vi "Vertex.vi"(4 "Radius":sgl=0.01, 5 "Font Size":sgl, 6 "Vertex label?":bool, 7 "Color":T1={"Red"=1.0, "Green"=0.0, "Blue"=0.0, "Alpha"=1.0}, 8 "error in (no error)":errorcluster, 9 "Length":sgl=2.0 step=0.01, 10 "Enum":enum16{"X Axis", "Y Axis", "Z Axis"}(ring), 11 "Name":string="XYZ axis") -> (0 "error out":errorcluster, 3 "New Object Refnum":refnum<vi>)   [LabVIEW 2021]
uses:
  <vilib>/Utility/miscctls.llb/LVSceneTextAlignment.ctl
  <vilib>/picture/3D Picture Control/Object/Create Object (name).vi
  <vilib>/picture/3D Picture Control/Object/Create Object (drawable).vi
  <vilib>/picture/3D Picture Control/Object/Add Object (no reference).vi
  <vilib>/picture/3D Picture Control/NI_3D Picture Control.lvlib
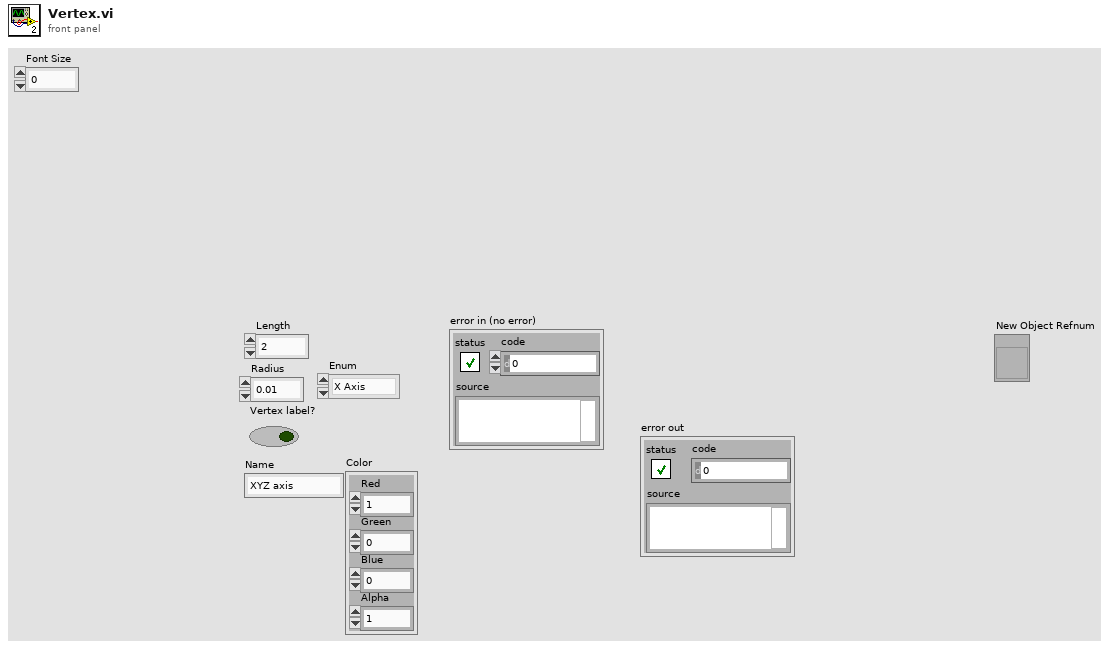
[diagram p1: front panel]
types:
  T1 = cluster{"Red":sgl, "Green":sgl, "Blue":sgl, "Alpha":sgl}
  T2 = typedef "LVSceneTextAlignment.ctl" = cluster{"Horizontal Alignment":enum8{"Left", "Right", "Center"}, "Vertical Alignment":enum8{"Top", "Bottom", "Center", "Base Line", "Bottom Base Line"}}
  T3 = cluster{"Alignment":T2, "Axis Alignment":enum8{"X-Y", "Y-Z", "X-Z", "Reversed X-Y", "Reversed Y-Z", "Reversed X-Z", "Screen"}, "Vertical?":bool, "Wrap Distance":sgl}
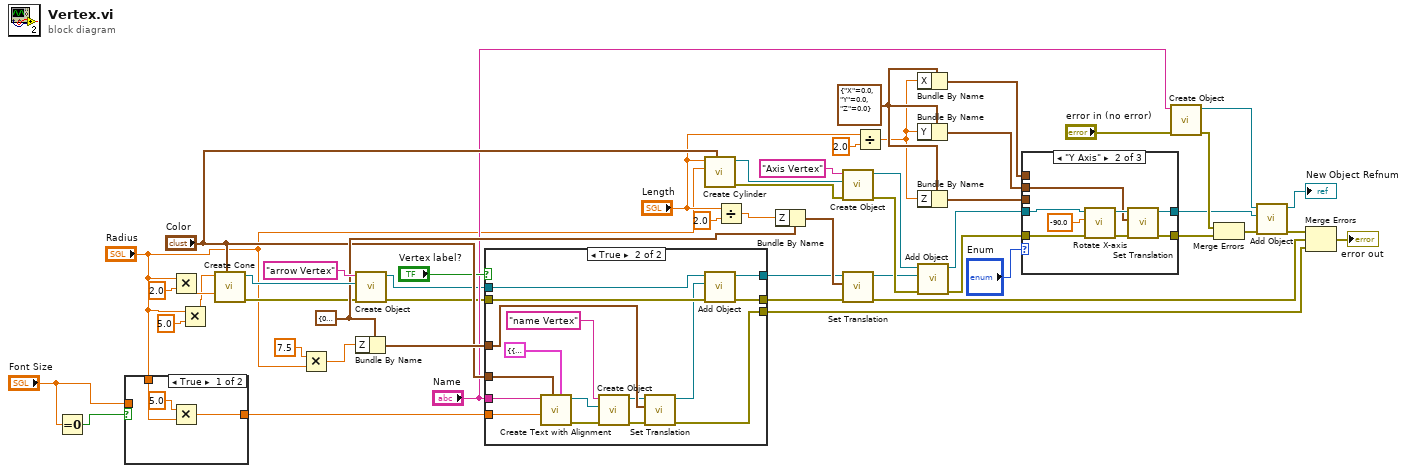
[diagram p0: block diagram]
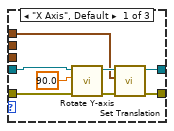
[diagram p3: hidden frame]
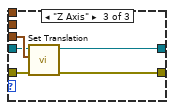
[diagram p4: hidden frame]
diagram:
  w40 = cluster{"X":sgl, "Y":sgl, "Z":sgl} {"X"=0.0, "Y"=0.0, "Z"=0.0} ("Translation")
  w38 = cluster{"X":sgl, "Y":sgl, "Z":sgl} {"X"=0.0, "Y"=0.0, "Z"=0.0} ("Translation")
  n1 = Equal To 0?(x="Font Size") -> (x = 0?=w5:bool)
  n2 = case shown="True" w5 {
    tunnel: "Radius" -> [w54 _]
    tunnel: [w53 w56] -> w7
    tunnel: "Font Size" -> [_ w56]
    frame True {
      n3 = Multiply(x=sgl 5.0 ("y"), y=w54) -> (x*y=w53:sgl)
    }
    frame False {
    }
  }
  n4 = Multiply(x="Radius", y=sgl 2.0) -> (x*y=w4:sgl)
  n5 = Multiply(x="Radius", y=sgl 5.0) -> (x*y=w1:sgl)
  n6 = call <vilib>:"Create Cone.vi"("Color"="Color", "Radius"=w4, "Height"=w1) -> ("error out"=w36:errorcluster, "New Cone Refnum"=w41:refnum<vi>)  [unwired: 7 in]
  n7 = Multiply(x=sgl 7.5 ("y"), y="Radius") -> (x*y=w8:sgl)
  n8 = call-poly <vilib>:"Create Object.vi"("error in (no error)"=w36, "Geometry"=w41, "Name"="arrow Vertex") -> ("error out"=w11:errorcluster, "Scene:New Object"=w10:refnum<vi>)  [unwired: 7 in]
  n9 = Bundle By Name(cluster=w38, "Z"=w8) -> (w37:cluster{"X":sgl, "Y":sgl, "Z":sgl})
  n10 = case shown="True" "Vertex label?" {
    tunnel: [w58 w74] -> w14
    tunnel: w37 -> [_ w73]
    tunnel: [w57 w72] -> w13
    tunnel: [_ w65] -> w28
    tunnel: "Color" -> [_ w71]
    tunnel: w7 -> [_ w66]
    tunnel: "Name" -> [_ w64]
    tunnel: w11 -> [w57 w62]
    tunnel: w10 -> [w58 w61]
    frame False {
    }
    frame True {
      n11 = call <vilib>:"Create Text with Alignment.vi"("Font Options"=T3 {"Alignment"={"Horizontal Alignment"=enum."Center", "Vertical Alignment"=enum."Center"}, "Axis Alignment"=enum."Screen", "Vertical?"=FALSE, "Wrap Distance"=0.0} ("Font options"), "Color"=w71, "Character Size"=w66, "Text"=w64) -> ("error out"=w67:errorcluster, "New Text Refnum"=w70:refnum<vi>)  [unwired: 6 in]
      n12 = call-poly <vilib>:"Create Object.vi"("error in (no error)"=w67, "Geometry"=w70, "Name"="name Vertex") -> ("error out"=w68:errorcluster, "Scene:New Object"=w69:refnum<vi>)  [unwired: 7 in]
      n13 = call <vilib>:"Set Translation.vi"("error in (no error)"=w68, "Translation"=w73, "Scene Object"=w69) -> ("error out"=w65:errorcluster, "Translated Object"=w60:refnum<vi>)  [unwired: 7 in]
      n14 = call-poly <vilib>:"Add Object.vi"("error in (no error)"=w62, "New Object In"=w60, "Scene Object In"=w61) -> ("error out"=w72:errorcluster, "Scene Object Out"=w74:refnum<vi>)  [unwired: 7 in]
    }
  }
  n15 = call <vilib>:"Create Cylinder.vi"("Color"="Color", "Radius"="Radius", "Height"="Length") -> ("error out"=w48:errorcluster, "New Cylinder Refnum"=w51:refnum<vi>)  [unwired: 7 in]
  n16 = Divide(x="Length", y=sgl 2.0 ("x")) -> (x/y=w35:sgl)
  n17 = Bundle By Name(cluster=w38, "Z"=w35) -> (w16:cluster{"X":sgl, "Y":sgl, "Z":sgl})
  n18 = call-poly <vilib>:"Create Object.vi"("error in (no error)"=w48, "Geometry"=w51, "Name"="Axis Vertex") -> ("error out"=w22:errorcluster, "Scene:New Object"=w21:refnum<vi>)  [unwired: 7 in]
  n19 = call <vilib>:"Set Translation.vi"("error in (no error)"=w13, "Translation"=w16, "Scene Object"=w14) -> ("error out"=w12:errorcluster, "Translated Object"=w15:refnum<vi>)  [unwired: 7 in]
  n20 = Divide(x="Length", y=sgl 2.0) -> (x/y=w39:sgl)
  n21 = Bundle By Name(cluster=w40, "X"=w39) -> (w32:cluster{"X":sgl, "Y":sgl, "Z":sgl})
  n22 = Bundle By Name(cluster=w40, "Y"=w39) -> (w25:cluster{"X":sgl, "Y":sgl, "Z":sgl})
  n23 = Bundle By Name(cluster=w40, "Z"=w39) -> (w24:cluster{"X":sgl, "Y":sgl, "Z":sgl})
  n24 = call-poly <vilib>:"Add Object.vi"("error in (no error)"=w22, "New Object In"=w15, "Scene Object In"=w21) -> ("error out"=w20:errorcluster, "Scene Object Out"=w19:refnum<vi>)  [unwired: 7 in]
  n25 = case shown="\"Y Axis\"" "Enum" {
    tunnel: w32 -> [w75 _ _]
    tunnel: [w76 w87 w93] -> w31
    tunnel: [w77 w86 w94] -> w30
    tunnel: w25 -> [_ w83 _]
    tunnel: w24 -> [_ _ w95]
    tunnel: w20 -> [w79 w85 w91]
    tunnel: w19 -> [w78 w84 w92]
    frame "X Axis", Default {
      n26 = call <vilib>:"Rotate Y-axis.vi"("error in (no error)"=w79, "angle"=90.0, "Scene Object In"=w78) -> ("error out"=w82:errorcluster, "Scene Object Out"=w81:refnum<vi>)  [unwired: 7 in]
      n27 = call <vilib>:"Set Translation.vi"("error in (no error)"=w82, "Translation"=w75, "Scene Object"=w81) -> ("error out"=w76:errorcluster, "Translated Object"=w77:refnum<vi>)  [unwired: 7 in]
    }
    frame "Y Axis" {
      n28 = call <vilib>:"Rotate X-axis.vi"("error in (no error)"=w85, "angle"=-90.0, "Scene Object In"=w84) -> ("error out"=w88:errorcluster, "Scene Object Out"=w89:refnum<vi>)  [unwired: 7 in]
      n29 = call <vilib>:"Set Translation.vi"("error in (no error)"=w88, "Translation"=w83, "Scene Object"=w89) -> ("error out"=w87:errorcluster, "Translated Object"=w86:refnum<vi>)  [unwired: 7 in]
    }
    frame "Z Axis" {
      n30 = call <vilib>:"Set Translation.vi"("error in (no error)"=w91, "Translation"=w95, "Scene Object"=w92) -> ("error out"=w93:errorcluster, "Translated Object"=w94:refnum<vi>)  [unwired: 7 in]
    }
  }
  n31 = call-poly <vilib>:"Create Object.vi"("error in (no error)"="error in (no error)", "Name"="Name") -> ("error out"=w47:errorcluster, "Scene:New Object"=w52:refnum<vi>)  [unwired: 8 in]
  n32 = Merge Errors(w47, w31) -> (w46:errorcluster)
  n33 = call-poly <vilib>:"Add Object.vi"("error in (no error)"=w46, "New Object In"=w30, "Scene Object In"=w52) -> ("error out"=w29:errorcluster, "Scene Object Out"=→"New Object Refnum":refnum<vi>)  [unwired: 7 in]
  n34 = Merge Errors(w29, w12, w28) -> (→"error out":errorcluster)
